vi "BuildMsgReportAnalogIOPin.vi"(8 "error in":errorcluster, 9 "Enable Continuous Reporting?":bool, 10 "Pin Index":u8 format="%x") -> (0 "error out":errorcluster, 2 "AnalogIOMessage":u8[](array[numeric]) format="%x", 4 "ReplyFirstByte":T1=224 items=["ANALOG_IO_MESSAGE"=224, "DIGITAL_IO_MESSAGE"=144, "REPORT_ANALOG_PIN"=192, "REPORT_DIGITAL_PORT"=208, "START_SYSEX"=240, "END_SYSEX"=247, "SET_PIN_MODE"=244, "SET_DIGITAL_PIN_VALUE"=245, "PROTOCOL_VERSION"=249, "SYSTEM_RESET"=255, "SYSEX.EXTENDED_ID"=0, "SYSEX.RESERVED_USER_COMMANDs"=1, "SYSEX.ANALOG_MAPPING_QUERY"=105, "SYSEX.ANALOG_MAPPING_RESPONSE"=106, "SYSEX.CAPABILITY_QUERY"=107, "SYSEX.CAPABILITY_RESPONSE"=108, "SYSEX.PIN_STATE_QUERY"=109, "SYSEX.PIN_STATE_RESPONSE"=110, "SYSEX.REPORT_FIRMWARE"=121, "SYSEX.EXTENDED_ANALOG"=111, "SYSEX.STRING_DATA"=113, "SYSEX.REALTIME"=127, "SYSEX.NON_REALTIME"=126, "SYSEX.SAMPLING_INTERVAL"=122, "FEATURES.SYSEX.I2C_READ_WRITE"=118, "FEATURES.SYSEX.I2C_REPLY"=119, "FEATURES.SYSEX.I2C_CONFIG"=120], 6 "ReplyLength":i32=-1)   [LabVIEW 2020, in "FirmataClient.lvlib"]
doc: "This message will enable / disable continuous report of a specific analog pin, by sending the \"Report Analog Pin\" message and expect the \"Analog IO Message\" as a reply.\n\nBuilds the message according to the Firmata Protocol Requirements. \n- https://github.com/firmata/protocol\n- https://github.com/firmata/protocol/blob/master/protocol.md"
uses:
  FirmataClient.lvlib
  Controls/FirmataProtocolConstants.ctl
  1a5eda8d-a658-419a-931f-f9d1827bf5cc.vi
  Utils/8BitsChar To 7bitsTokens.vi
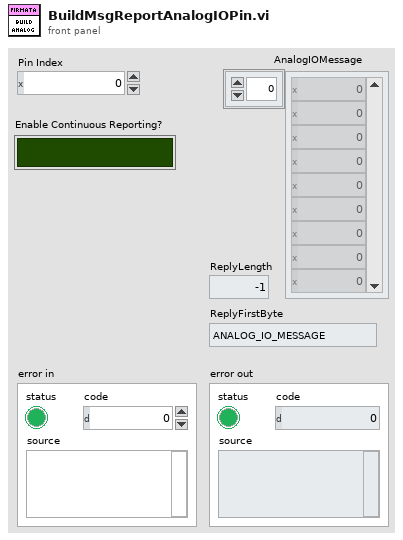
[diagram p1: front panel]
types:
  T1 = typedef "FirmataClient.lvlib/FirmataProtocolConstants.ctl" = u16
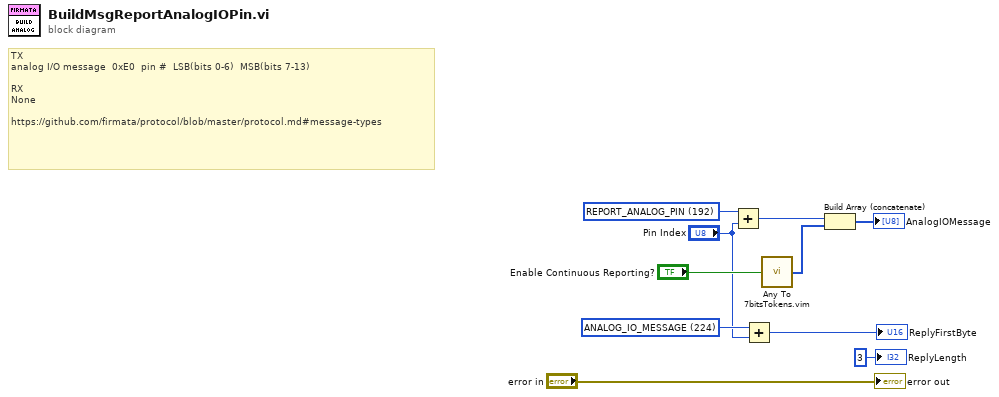
[diagram p0: block diagram]
diagram:
  w3 = T1 224 items=["ANALOG_IO_MESSAGE"=224, "DIGITAL_IO_MESSAGE"=144, "REPORT_ANALOG_PIN"=192, "REPORT_DIGITAL_PORT"=208, "START_SYSEX"=240, "END_SYSEX"=247, "SET_PIN_MODE"=244, "SET_DIGITAL_PIN_VALUE"=245, "PROTOCOL_VERSION"=249, "SYSTEM_RESET"=255, "SYSEX.EXTENDED_ID"=0, "SYSEX.RESERVED_USER_COMMANDs"=1, "SYSEX.ANALOG_MAPPING_QUERY"=105, "SYSEX.ANALOG_MAPPING_RESPONSE"=106, "SYSEX.CAPABILITY_QUERY"=107, "SYSEX.CAPABILITY_RESPONSE"=108, "SYSEX.PIN_STATE_QUERY"=109, "SYSEX.PIN_STATE_RESPONSE"=110, "SYSEX.REPORT_FIRMWARE"=121, "SYSEX.EXTENDED_ANALOG"=111, "SYSEX.STRING_DATA"=113, "SYSEX.REALTIME"=127, "SYSEX.NON_REALTIME"=126, "SYSEX.SAMPLING_INTERVAL"=122, "FEATURES.SYSEX.I2C_READ_WRITE"=118, "FEATURES.SYSEX.I2C_REPLY"=119, "FEATURES.SYSEX.I2C_CONFIG"=120] ("FimataProtocolConstants")
  w7 = T1 192 items=["ANALOG_IO_MESSAGE"=224, "DIGITAL_IO_MESSAGE"=144, "REPORT_ANALOG_PIN"=192, "REPORT_DIGITAL_PORT"=208, "START_SYSEX"=240, "END_SYSEX"=247, "SET_PIN_MODE"=244, "SET_DIGITAL_PIN_VALUE"=245, "PROTOCOL_VERSION"=249, "SYSTEM_RESET"=255, "SYSEX.EXTENDED_ID"=0, "SYSEX.RESERVED_USER_COMMANDs"=1, "SYSEX.ANALOG_MAPPING_QUERY"=105, "SYSEX.ANALOG_MAPPING_RESPONSE"=106, "SYSEX.CAPABILITY_QUERY"=107, "SYSEX.CAPABILITY_RESPONSE"=108, "SYSEX.PIN_STATE_QUERY"=109, "SYSEX.PIN_STATE_RESPONSE"=110, "SYSEX.REPORT_FIRMWARE"=121, "SYSEX.EXTENDED_ANALOG"=111, "SYSEX.STRING_DATA"=113, "SYSEX.REALTIME"=127, "SYSEX.NON_REALTIME"=126, "SYSEX.SAMPLING_INTERVAL"=122, "FEATURES.SYSEX.I2C_READ_WRITE"=118, "FEATURES.SYSEX.I2C_REPLY"=119, "FEATURES.SYSEX.I2C_CONFIG"=120] ("FimataProtocolConstants")
  # "TX\nanalog I/O message \t0xE0 \tpin # \tLSB(bits 0-6) \tMSB(bits 7-13)\n\nRX\nNone\n\nhttps://github.com/firmata/protocol/blob/master/protocol.md#message-types"
  n1 = Add(x=w7, y="Pin Index") -> (x+y=w9:T1)
  n2 = Add(x=w3, y="Pin Index") -> (x+y=→"ReplyFirstByte":T1)
  n3 = call "Any To 7bitsTokens.vim"("Byte In"="Enable Continuous Reporting?") -> ("Byte Out"=w6:u32[])
  n4 = Build Array (concatenate)(w9, w6) -> (→"AnalogIOMessage":u32[])
  "error out" <- "error in"
  "ReplyLength" <- 3 ("ReplyLength")
